vi "utility_bgk_3475.vi"(8 "error in":errorcluster caption="错误输入（无错误）", 11 "VISA resource name":refnum<visa-resource-name>="COM2") -> (0 "error out":errorcluster caption="错误输出")   [LabVIEW 2015]
uses:
  <vilib>/Instr/_visa.llb/VISA Configure Serial Port (Instr).vi
panel:
  out "read from buffer":string caption="读取缓冲区"
  out "valid reply?":bool caption="合法回复?"
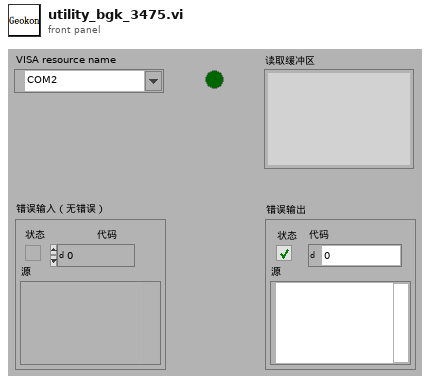
[diagram p1: front panel]
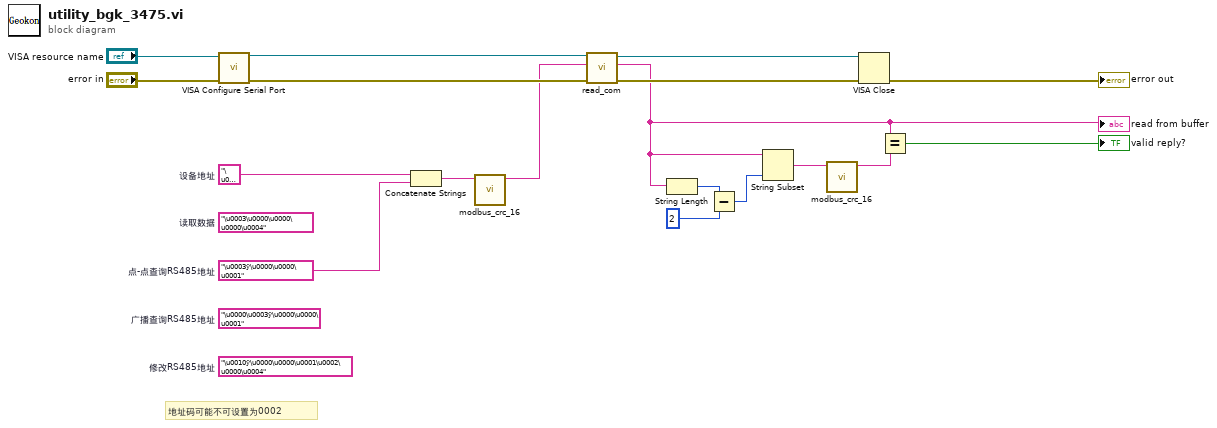
[diagram p0: block diagram]
diagram:
  (unwired) "\u0010ÿ\u0000\u0000\u0001\u0002\u0000\u0004"  # 修改RS485地址
  (unwired) "\u0000\u0003ÿ\u0000\u0000\u0001"  # 广播查询RS485地址
  w1 = "\u0003ÿ\u0000\u0000\u0001"  # 点-点查询RS485地址
  w3 = "\u0004"  # 设备地址
  (unwired) "\u0003\u0000\u0000\u0000\u0004"  # 读取数据
  # "地址码可能不可设置为0002"
  n1 = call-poly "VISA Configure Serial Port"("VISA resource name"="VISA resource name", "error in (no error)"="error in") -> ("VISA resource name out"=w16:refnum<visa-resource-name>, "error out"=w15:errorcluster)  [unwired: 12 in]
  n2 = Concatenate Strings(w3, w1) -> (w10:string)
  n3 = call "modbus_crc_16.vi"("String"=w10) -> ("String & CRC-16"=w11:string)  [unwired: 9 in, 1 out]
  n4 = call "read_com.vi"("error in"=w15, "write to buffer"=w11, "VISA resource name in"=w16) -> ("error out"=w17:errorcluster, "read from buffer"=w9:string, "VISA resource name out"=w18:refnum<visa-resource-name>)  [unwired: 5 in, 1 out]
  "read from buffer" <- w9
  n5 = String Length(string=w9) -> (length=w6:i32)
  n6 = Subtract(x=w6, y=2) -> (x-y=w5:i32)
  n7 = String Subset(string=w9, length (rest)=w5) -> (substring=w7:string)  [unwired: 1 in]
  n8 = call "modbus_crc_16.vi"("String"=w7) -> ("String & CRC-16"=w8:string)  [unwired: 9 in, 1 out]
  n9 = VISA Close(VISA resource name=w18, error in (no error)=w17) -> (error out=→"error out":errorcluster)
  n10 = Equal?(x=w9, y=w8) -> (x = y?=→"valid reply?":bool)
